vi "FooBar.vi"() -> ()   [LabVIEW 2015]
panel:
  in  "DAQ Channel To Read":refnum<k21>
  out "error out":errorcluster
  out "State":bool
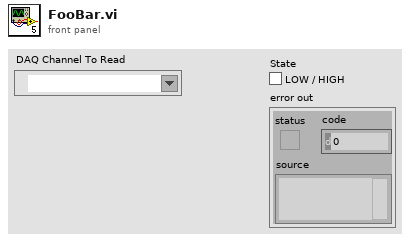
[diagram p1: front panel]
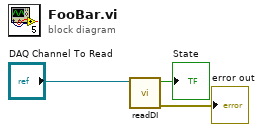
[diagram p0: block diagram]
diagram:
  n1 = call <userlib>:"readDI.vi"("DAQ Channel To Read"="DAQ Channel To Read") -> ("error out"=→"error out":errorcluster, "State"=→"State":bool)  [unwired: 9 in]
